vi "LineScanCounterAE.vi"(5 "# Accumulated (reference)":refnum<vi>, 7 "Current point index (reference)":refnum<vi>, 9 "Number of points":i32=2, 10 "Accumulate to #":i32=2, 11 "Task":T1) -> (0 "Line completed":bool, 1 "Done with point":bool, 2 "# Accumulated":i32, 3 "Current point index":i32, 4 "Number of points (query)":i32, 6 "Accumulate to (query)":i32, 8 "Active":bool)   [LabVIEW 2022 SP3]
uses:
  Control_LineScanCounterAE.ctl
panel:
  out "Completed":bool
  out "Ultimate point":bool
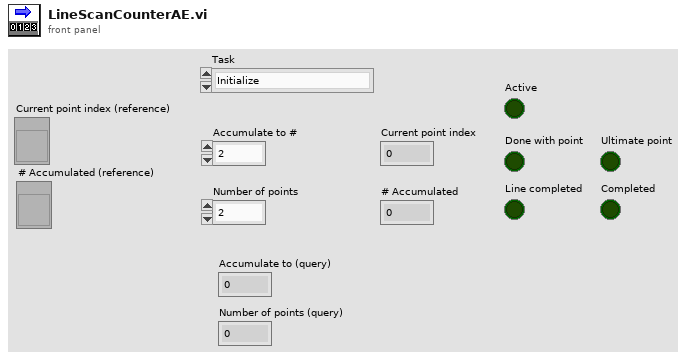
[diagram p1: front panel]
types:
  T1 = typedef "Control_LineScanCounterAE.ctl" = enum16{"Initialize", "Activate", "Attach indicators", "Increment Point", "Query", "Do Finish Point", "Acknowledge line", "Deactivate"}
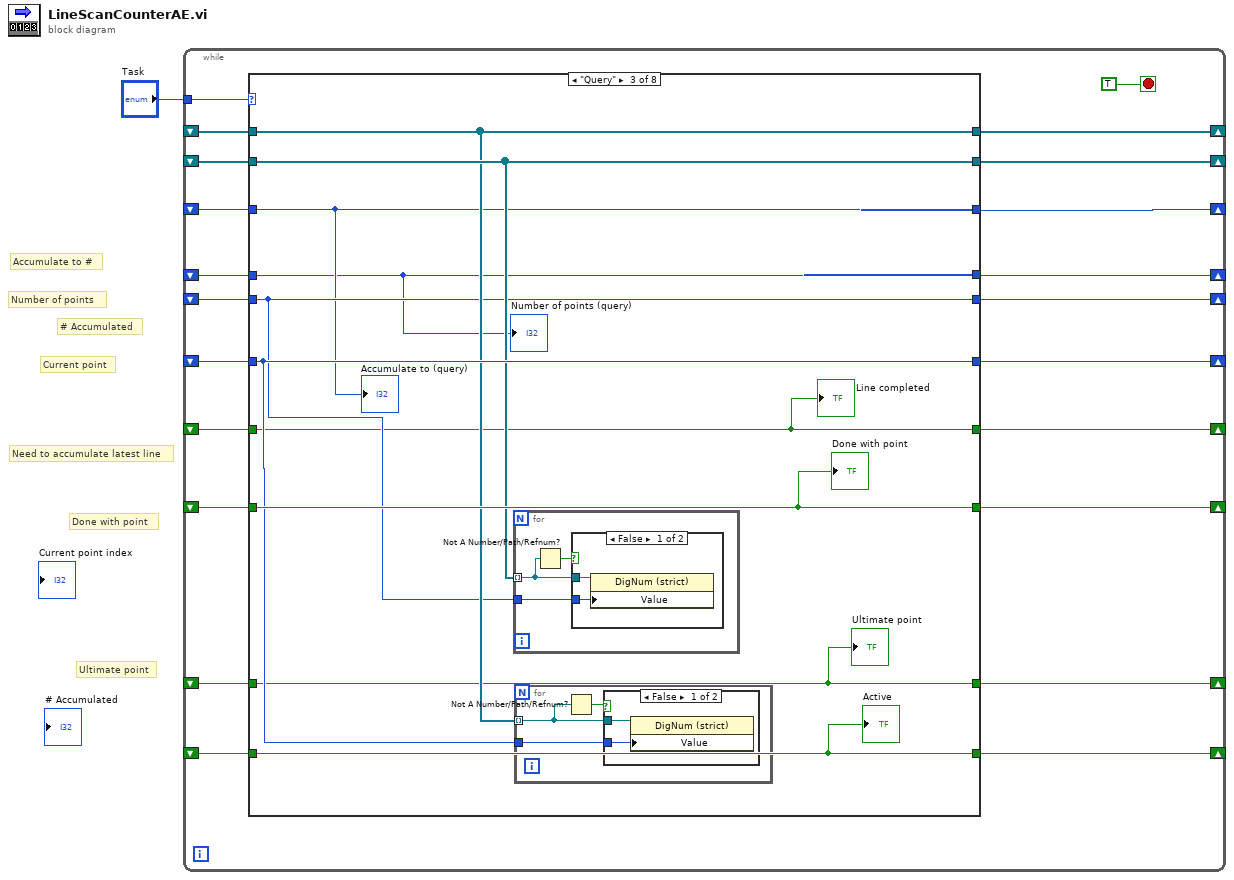
[diagram p0: block diagram]
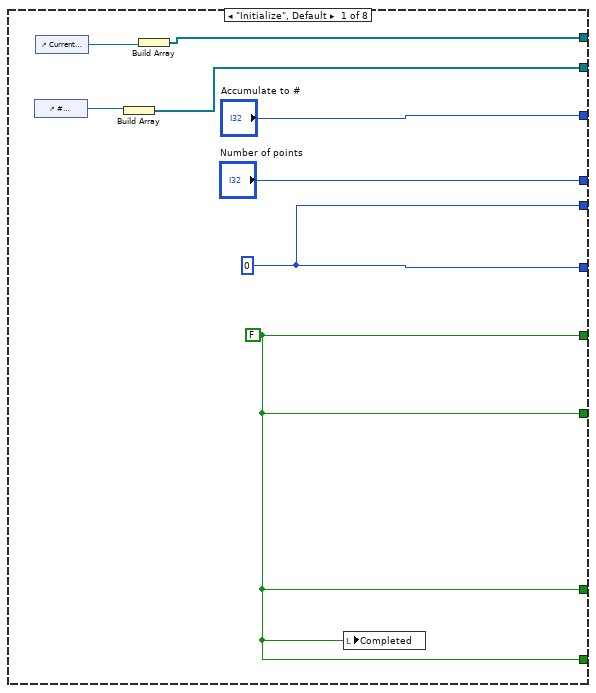
[diagram p2: hidden frame]
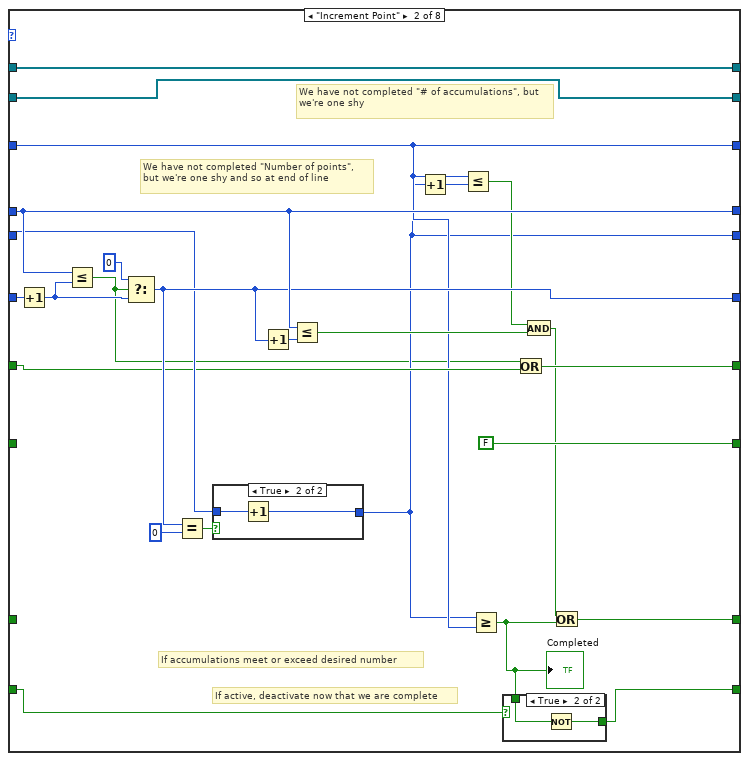
[diagram p3: hidden frame]
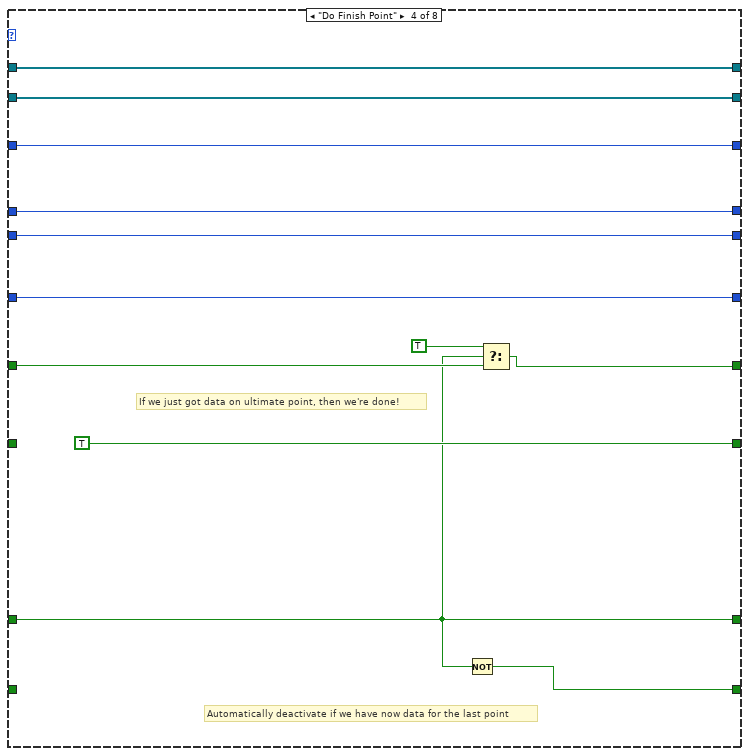
[diagram p8: hidden frame]
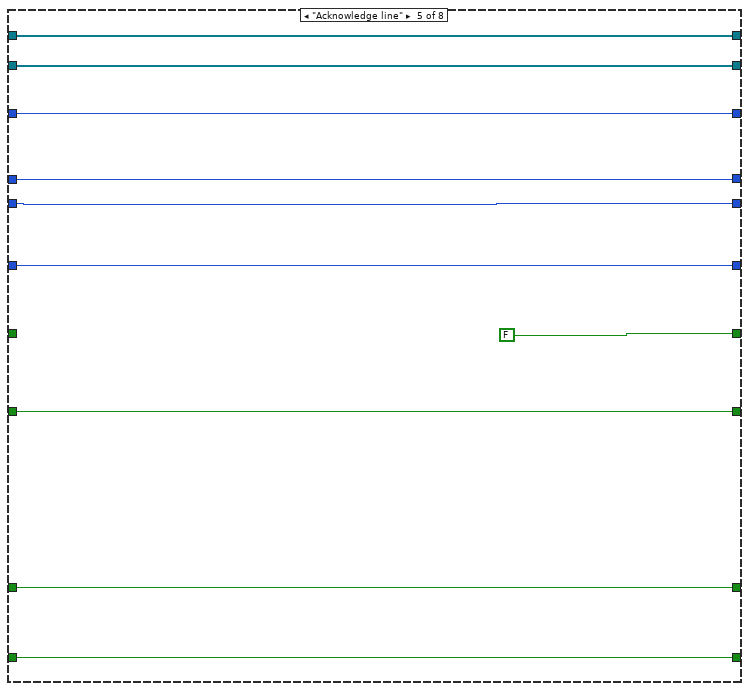
[diagram p9: hidden frame]
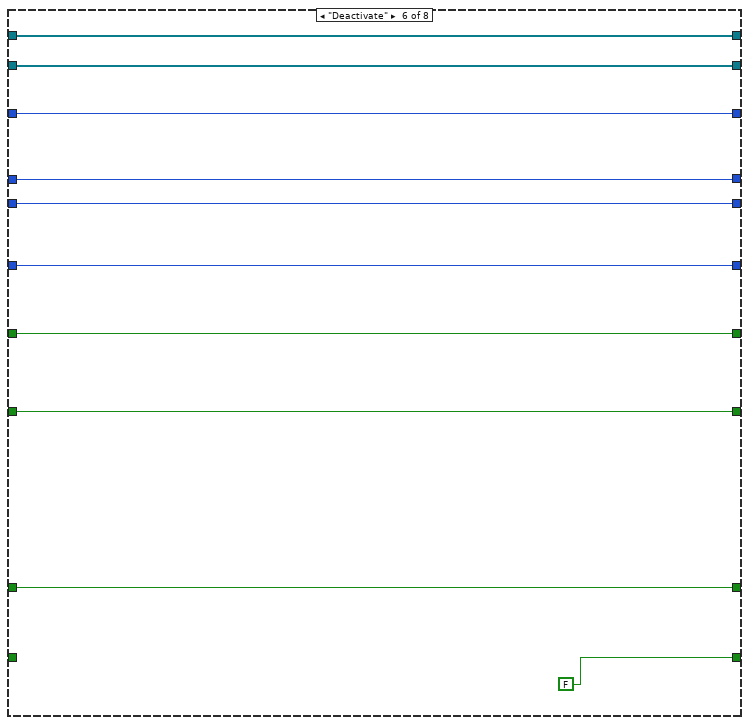
[diagram p10: hidden frame]
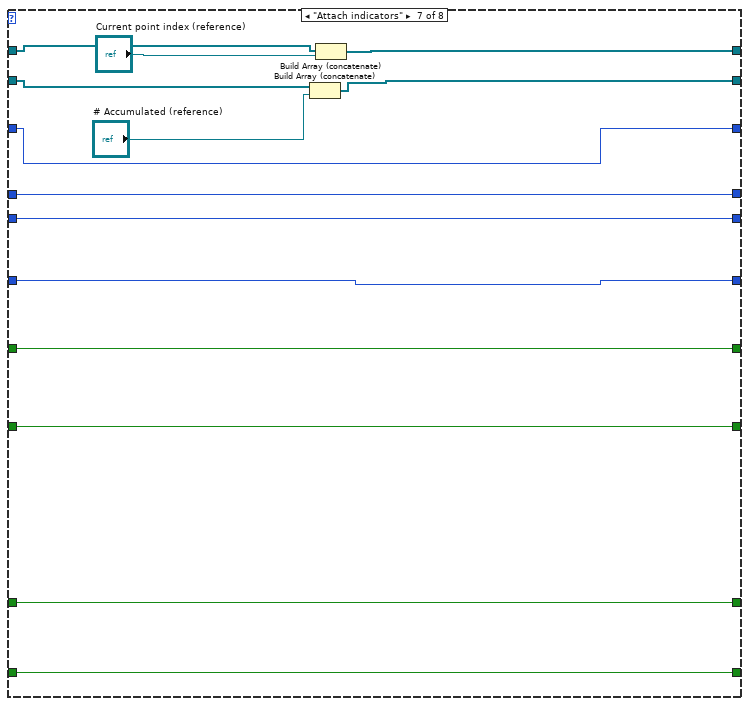
[diagram p11: hidden frame]
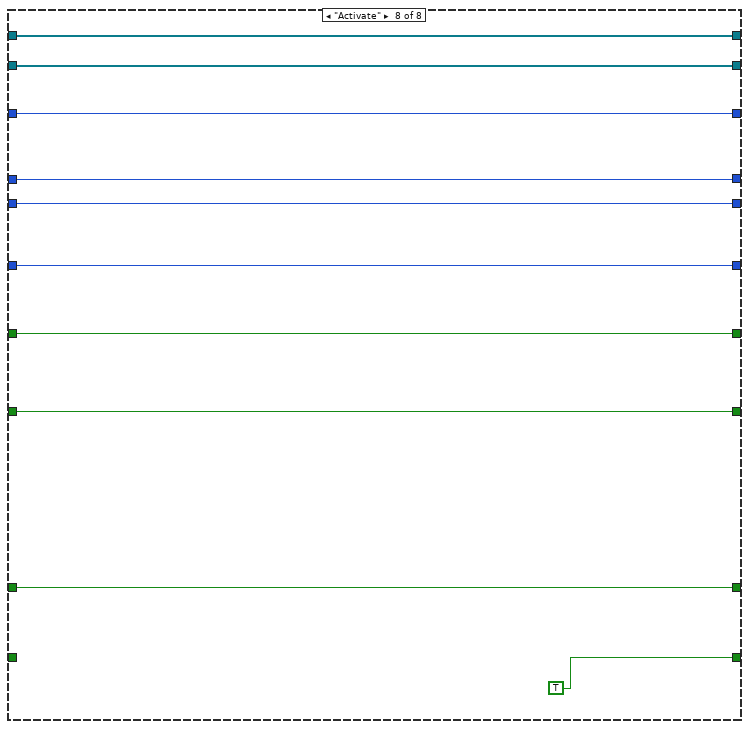
[diagram p12: hidden frame]
diagram:
  # "# Accumulated"
  # "Ultimate point"
  # "Done with point"
  # "Need to accumulate latest line"
  # "Current point"
  # "Accumulate to #"
  # "Number of points"
  n1 = while {
    tunnel: "Task" -> [w23]
    shift-right: [w21] -> _
    shift-left: _ -> [w18]
    shift-right: [w22] -> _
    shift-left: _ -> [w19]
    shift-right: [w2] -> _
    shift-left: _ -> [w17]
    shift-right: [w16] -> _
    shift-left: _ -> [w15]
    shift-right: [w4] -> _
    shift-left: _ -> [w14]
    shift-right: [w13] -> _
    shift-left: _ -> [w12]
    shift-right: [w11] -> _
    shift-left: _ -> [w10]
    shift-right: [w3] -> _
    shift-left: _ -> [w9]
    shift-right: [w5] -> _
    shift-left: _ -> [w8]
    shift-right: [w7] -> _
    shift-left: _ -> [w6]
    stop <- TRUE stop-if-true
    n2 = case shown="\"Query\"" w23 {
      tunnel: ["Accumulate to #" w37 w66 w89 w101 w107 w128 w135] -> w22
      tunnel: ["Number of points" w51 w65 w88 w100 w108 w127 w134] -> w21
      tunnel: w19 -> [_ w37 w66 w89 w101 w107 w128 w135]
      tunnel: w18 -> [_ w51 w65 w88 w100 w108 w127 w134]
      tunnel: [w29 w49 w71 w93 w104 w110 w120 w132] -> w2
      tunnel: w17 -> [_ w56 w71 w93 w104 w110 w120 w132]
      tunnel: [w24 w42 w64 w83 FALSE w111 w126 w131] -> w16
      tunnel: w15 -> [_ w40 w64 w86 _ w111 w126 w131]
      tunnel: [w29 w36 w68 w92 w96 w109 w122 w133] -> w4
      tunnel: w14 -> [_ w47 w68 w92 w96 w109 w122 w133]
      tunnel: [w24 FALSE w72 TRUE w103 w112 w125 w130] -> w13
      tunnel: w12 -> [_ _ w72 _ w103 w112 w125 w130]
      tunnel: [w24 w38 w63 w85 w98 w113 w124 w129] -> w11
      tunnel: w10 -> [_ _ w63 w85 w98 w113 w124 w129]
      tunnel: [w28 w45 w69 w91 w102 w105 w119 w137] -> w3
      tunnel: [w27 w46 w70 w90 w99 w106 w121 w136] -> w5
      tunnel: w9 -> [_ w45 w69 w91 w102 w105 w117 w137]
      tunnel: w8 -> [_ w46 w70 w90 w99 w106 w116 w136]
      tunnel: [w24 w33 w67 w87 w95 FALSE w123 TRUE] -> w7
      tunnel: w6 -> [_ w35 w67 _ w95 _ w123 _]
      frame "Initialize", Default {
        w24 = FALSE
        w29 = 0
        n3 = control-ref of="# Accumulated"() -> (w25:refnum<vi>)
        n4 = control-ref of="Current point index"() -> (w26:refnum<vi>)
        n5 = Build Array(w25) -> (w27:refnum<vi>[])
        n6 = Build Array(w26) -> (w28:refnum<vi>[])
        n7 = local write "Completed"(w24) -> ()
      }
      frame "Increment Point" {
        # "If active, deactivate now that we are complete"
        # "If accumulations meet or exceed desired number"
        # "We have not completed \"# of accumulations\", but we're one shy"
        # "We have not completed \"Number of points\", but we're one shy and so at end of line"
        n8 = Increment(x=w56) -> (x+1=w55:i32)
        n9 = Less Or Equal?(x=w51, y=w55) -> (x <= y?=w32:bool)
        n10 = Select(t=0, s=w32, f=w55) -> (s? t:f=w49:i32)
        n11 = Equal?(x=w49, y=0) -> (x = y?=w48:bool)
        n12 = case shown="True" w48 {
          tunnel: w47 -> [w60 w62]
          tunnel: [w60 w61] -> w36
          frame False {
          }
          frame True {
            n13 = Increment(x=w62) -> (x+1=w61:i32)
          }
        }
        n14 = Increment(x=w49) -> (x+1=w52:i32)
        n15 = Less Or Equal?(x=w51, y=w52) -> (x <= y?=w41:bool)
        n16 = Increment(x=w36) -> (x+1=w44:i32)
        n17 = Less Or Equal?(x=w37, y=w44) -> (x <= y?=w43:bool)
        n18 = Greater Or Equal?(x=w36, y=w37) -> (x >= y?=w34:bool)
        "Completed" <- w34
        n19 = case shown="True" w35 {
          selector: w35 -> [w57 _]
          tunnel: w34 -> [_ w59]
          tunnel: [w57 w58] -> w33
          frame False {
          }
          frame True {
            n20 = Not(x=w59) -> (.not. x?=w58:bool)
          }
        }
        n21 = Or(x=w32, y=w40) -> (x .or. y?=w42:bool)
        n22 = And(x=w43, y=w41) -> (x .and. y?=w39:bool)
        n23 = Or(x=w39, y=w34) -> (x .or. y?=w38:bool)
      }
      frame "Query" {
        n24 = for {
          tunnel: w68 -> [w80]
          tunnel: w70 -> [w79] mode=indexing
          n25 = Not A Number/Path/Refnum?(number/path/refnum=w79) -> (NaN/Path/Refnum?=w78:bool)
          n26 = case shown="False" w78 {
            tunnel: w80 -> [w82 _]
            tunnel: w79 -> [w81 _]
            frame False {
              n27 = property on="Property Node" class="DigNum (strict)"(reference=w81, "Value"=w82) -> ()  [unwired: 1 in, 2 out]
            }
            frame True {
            }
          }
        }
        n28 = for {
          tunnel: w71 -> [w75]
          tunnel: w69 -> [w74] mode=indexing
          n29 = Not A Number/Path/Refnum?(number/path/refnum=w74) -> (NaN/Path/Refnum?=w73:bool)
          n30 = case shown="False" w73 {
            tunnel: w75 -> [w77 _]
            tunnel: w74 -> [w76 _]
            frame False {
              n31 = property on="Property Node" class="DigNum (strict)"(reference=w76, "Value"=w77) -> ()  [unwired: 1 in, 2 out]
            }
            frame True {
            }
          }
        }
        "Accumulate to (query)" <- w66
        "Number of points (query)" <- w65
        "Line completed" <- w64
        "Done with point" <- w72
        "Ultimate point" <- w63
        "Active" <- w67
      }
      frame "Do Finish Point" {
        # "If we just got data on ultimate point, then we're done!"
        # "Automatically deactivate if we have now data for the last point"
        n32 = Not(x=w85) -> (.not. x?=w87:bool)
        n33 = Select(t=TRUE, s=w85, f=w86) -> (s? t:f=w83:bool)
      }
      frame "Acknowledge line" {
      }
      frame "Deactivate" {
      }
      frame "Attach indicators" {
        n34 = Build Array (concatenate)(w116, "# Accumulated (reference)") -> (w121:refnum<vi>[])
        n35 = Build Array (concatenate)(w117, "Current point index (reference)") -> (w119:refnum<vi>[])
      }
      frame "Activate" {
      }
    }
  }
